vi "LoadFileName_171213.vi"(11 "SelectedPath":path) -> (3 "FIleName":string)   [LabVIEW 2016]
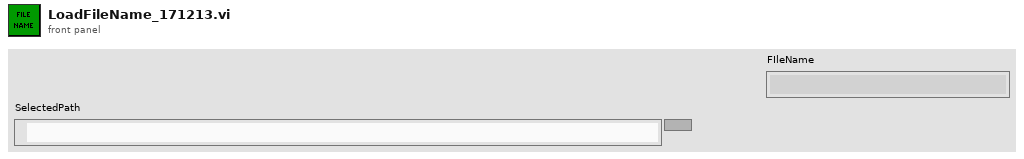
[diagram p1: front panel]
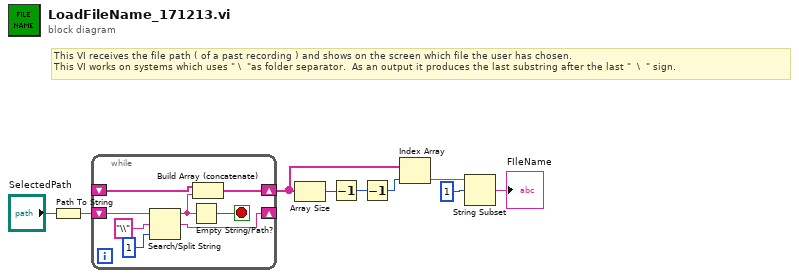
[diagram p0: block diagram]
diagram:
  # "This VI receives the file path ( of a past recording ) and shows on the screen which file the user has chosen.\nThis VI works on systems which uses \" \\  \"as folder separator.  As an output it produces the last substring after the last \"  \\  \" sign."
  n1 = Path To String(path="SelectedPath") -> (string=w8:string)
  n2 = while {
    shift-right: [w17] -> _
    shift-left: w8 -> [w11]
    shift-right: [w15] -> w6
    shift-left: _ -> [w14]
    stop <- w12 stop-if-true
    n3 = Search/Split String(string=w11, search string/char (-)="\\", offset (0)=1) -> (substring before match=w13:string, match + rest of string=w17:string)  [unwired: 1 out]
    n4 = Empty String/Path?(string/path=w13) -> (empty?=w12:bool)
    n5 = Build Array (concatenate)(w14, w13) -> (w15:string[])
  }
  n6 = Array Size(array=w6) -> (size(s)=w7:i32)
  n7 = Decrement(x=w7) -> (x-1=w5:i32)
  n8 = Decrement(x=w5) -> (x-1=w4:i32)
  n9 = Index Array(array=w6, index=w4) -> (element=w3:string)
  n10 = String Subset(string=w3, offset (0)=1) -> (substring=→"FIleName":string)  [unwired: 1 in]
